vi "image analyze.vi"() -> ()   [LabVIEW 2017]
uses:
  <vilib>/httpClient/MultipartData.ctl
  <vilib>/httpClient/LabVIEWHTTPClient.lvlib
panel:
  out "Response":string
  in  "URL":string="http://192.168.0.100:8000/analyze_image"
  in  "Image path":path
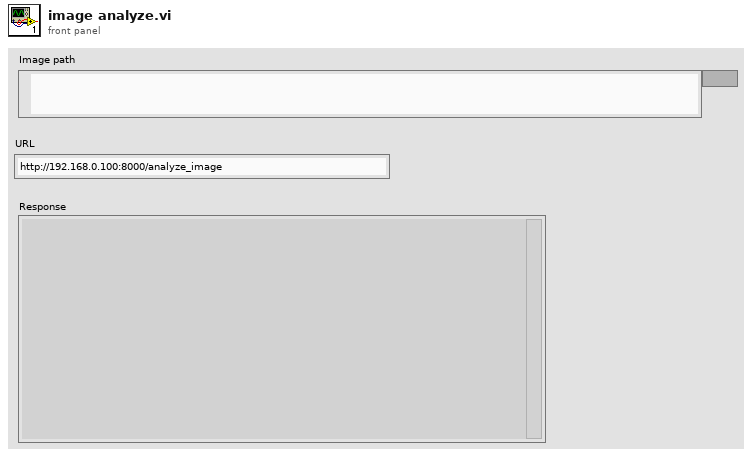
[diagram p1: front panel]
types:
  T1 = typedef "LabVIEWHTTPClient.lvlib/MultipartData.ctl" = cluster{"Name":string, "Value":string, "File":path, "Filename":string, "MIME type":string}
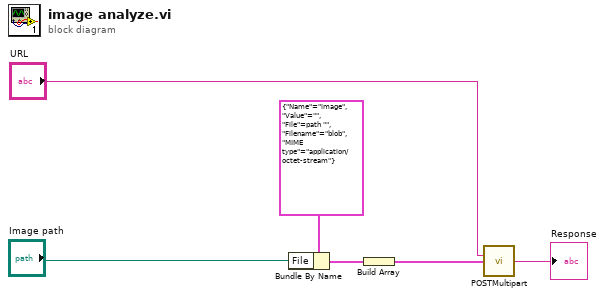
[diagram p0: block diagram]
diagram:
  n1 = Bundle By Name(cluster=T1 {"Name"="image", "Value"="", "File"=path "", "Filename"="blob", "MIME type"="application/octet-stream"} ("element"), "File"="Image path") -> (w4:T1)
  n2 = Build Array(w4) -> (w3:T1[])
  n3 = call <vilib>:"POSTMultipart.vi"("url"="URL", "data"=w3) -> ("body"=→"Response":string)  [unwired: 10 in, 3 out]
